vi "XX-孔数处理函数.vi"(0 "Image in":T2(plugin-control), 5 "参数输入":T1={"二值化参数"={"Lower value"=104.0, "Upper value"=255.0}, "Selection Values"=[{"Measurement Parameter"=35, "Range Lower Value"=1949.8375244140625, "Range Upper Value"=6069341.0, "Range"=FALSE, "Measurement Type"=FALSE}], "Selection Values2"=[{"Measurement Parameter"=19, "Range Lower Value"=98.7405776977539, "Range Upper Value"=135.92166137695312, "Range"=FALSE, "Measurement Type"=FALSE}]} {"Selection Values2"."Measurement Parameter" items=["Center of Mass X", "Center of Mass Y", "First Pixel X", "First Pixel Y", "Bounding Rect Left", "Bounding Rect Top", "Bounding Rect Right", "Bounding Rect Bottom", "Max Feret Diameter Start X", "Max Feret Diameter Start Y", "Max Feret Diameter End X", "Max Feret Diameter End Y", "Max Horiz. Segment Length Left", "Max Horiz. Segment Length Right", "Max Horiz. Segment Length Row", "-", "Bounding Rect Width", "Bounding Rect Height", "Bounding Rect Diagonal", "Perimeter", "Convex Hull Perimeter", "Holes' Perimeter", "Max Feret Diameter", "Equivalent Ellipse Major Axis", "Equivalent Ellipse Minor Axis", "Equivalent Ellipse Minor Axis (Feret)", "Equivalent Rect Long Side", "Equivalent Rect Short Side", "Equivalent Rect Diagonal", "Equivalent Rect Short Side (Feret)", "Average Horiz. Segment Length", "Average Vert. Segment Length", "Hydraulic Radius", "Waddel Disk Diameter", "-", "Area", "Holes' Area", "Particle & Holes' Area", "Convex Hull Area", "Image Area", "-", "Number of Holes", "Number of Horiz. Segments", "Number of Vert. Segments", "-", "Orientation", "Max Feret Diameter Orientation", "-", "% Area/Image Area", "% Area/(Particle & Holes' Area)", "Ratio of Equivalent Ellipse Axes", "Ratio of Equivalent Rect Sides", "-", "Elongation Factor", "Compactness Factor", "Heywood Circularity Factor", "Type Factor", "-", "Sum X", "Sum Y", "Sum XX", "Sum XY", "Sum YY", "Sum XXX", "Sum XXY", "Sum XYY", "Sum YYY", "-", "Moment of Inertia XX", "Moment of Inertia XY", "Moment of Inertia YY", "Moment of Inertia XXX", "Moment of Inertia XXY", "Moment of Inertia XYY", "Moment of Inertia YYY", "Norm. Moment of Inertia XX", "Norm. Moment of Inertia XY", "Norm. Moment of Inertia YY", "Norm. Moment of Inertia XXX", "Norm. Moment of Inertia XXY", "Norm. Moment of Inertia XYY", "Norm. Moment of Inertia YYY", "Hu Moment 1", "Hu Moment 2", "Hu Moment 3", "Hu Moment 4", "Hu Moment 5", "Hu Moment 6", "Hu Moment 7"]; "Selection Values"."Measurement Parameter" items=["Center of Mass X", "Center of Mass Y", "First Pixel X", "First Pixel Y", "Bounding Rect Left", "Bounding Rect Top", "Bounding Rect Right", "Bounding Rect Bottom", "Max Feret Diameter Start X", "Max Feret Diameter Start Y", "Max Feret Diameter End X", "Max Feret Diameter End Y", "Max Horiz. Segment Length Left", "Max Horiz. Segment Length Right", "Max Horiz. Segment Length Row", "-", "Bounding Rect Width", "Bounding Rect Height", "Bounding Rect Diagonal", "Perimeter", "Convex Hull Perimeter", "Holes' Perimeter", "Max Feret Diameter", "Equivalent Ellipse Major Axis", "Equivalent Ellipse Minor Axis", "Equivalent Ellipse Minor Axis (Feret)", "Equivalent Rect Long Side", "Equivalent Rect Short Side", "Equivalent Rect Diagonal", "Equivalent Rect Short Side (Feret)", "Average Horiz. Segment Length", "Average Vert. Segment Length", "Hydraulic Radius", "Waddel Disk Diameter", "-", "Area", "Holes' Area", "Particle & Holes' Area", "Convex Hull Area", "Image Area", "-", "Number of Holes", "Number of Horiz. Segments", "Number of Vert. Segments", "-", "Orientation", "Max Feret Diameter Orientation", "-", "% Area/Image Area", "% Area/(Particle & Holes' Area)", "Ratio of Equivalent Ellipse Axes", "Ratio of Equivalent Rect Sides", "-", "Elongation Factor", "Compactness Factor", "Heywood Circularity Factor", "Type Factor", "-", "Sum X", "Sum Y", "Sum XX", "Sum XY", "Sum YY", "Sum XXX", "Sum XXY", "Sum XYY", "Sum YYY", "-", "Moment of Inertia XX", "Moment of Inertia XY", "Moment of Inertia YY", "Moment of Inertia XXX", "Moment of Inertia XXY", "Moment of Inertia XYY", "Moment of Inertia YYY", "Norm. Moment of Inertia XX", "Norm. Moment of Inertia XY", "Norm. Moment of Inertia YY", "Norm. Moment of Inertia XXX", "Norm. Moment of Inertia XXY", "Norm. Moment of Inertia XYY", "Norm. Moment of Inertia YYY", "Hu Moment 1", "Hu Moment 2", "Hu Moment 3", "Hu Moment 4", "Hu Moment 5", "Hu Moment 6", "Hu Moment 7"]; "Selection Values"."Range Upper Value" format="%#_9f"}, 7 "图像处理开关":bool, 11 "error in":errorcluster) -> (4 "Image Out":T2(plugin-control), 10 "Particle Measurements (Pixels)":dbl[][](array[numeric]) format="%.2f", 15 "error out":errorcluster)   [LabVIEW 2017]
uses:
  Global System.vi
  <vilib>/vision/NI_Vision_Development_Module.lvlib
panel:
  out "millisecond timer value":u32
  in  "Range":cluster{"Lower value":sgl, "Upper value":sgl}={"Lower value"=104.0, "Upper value"=255.0}
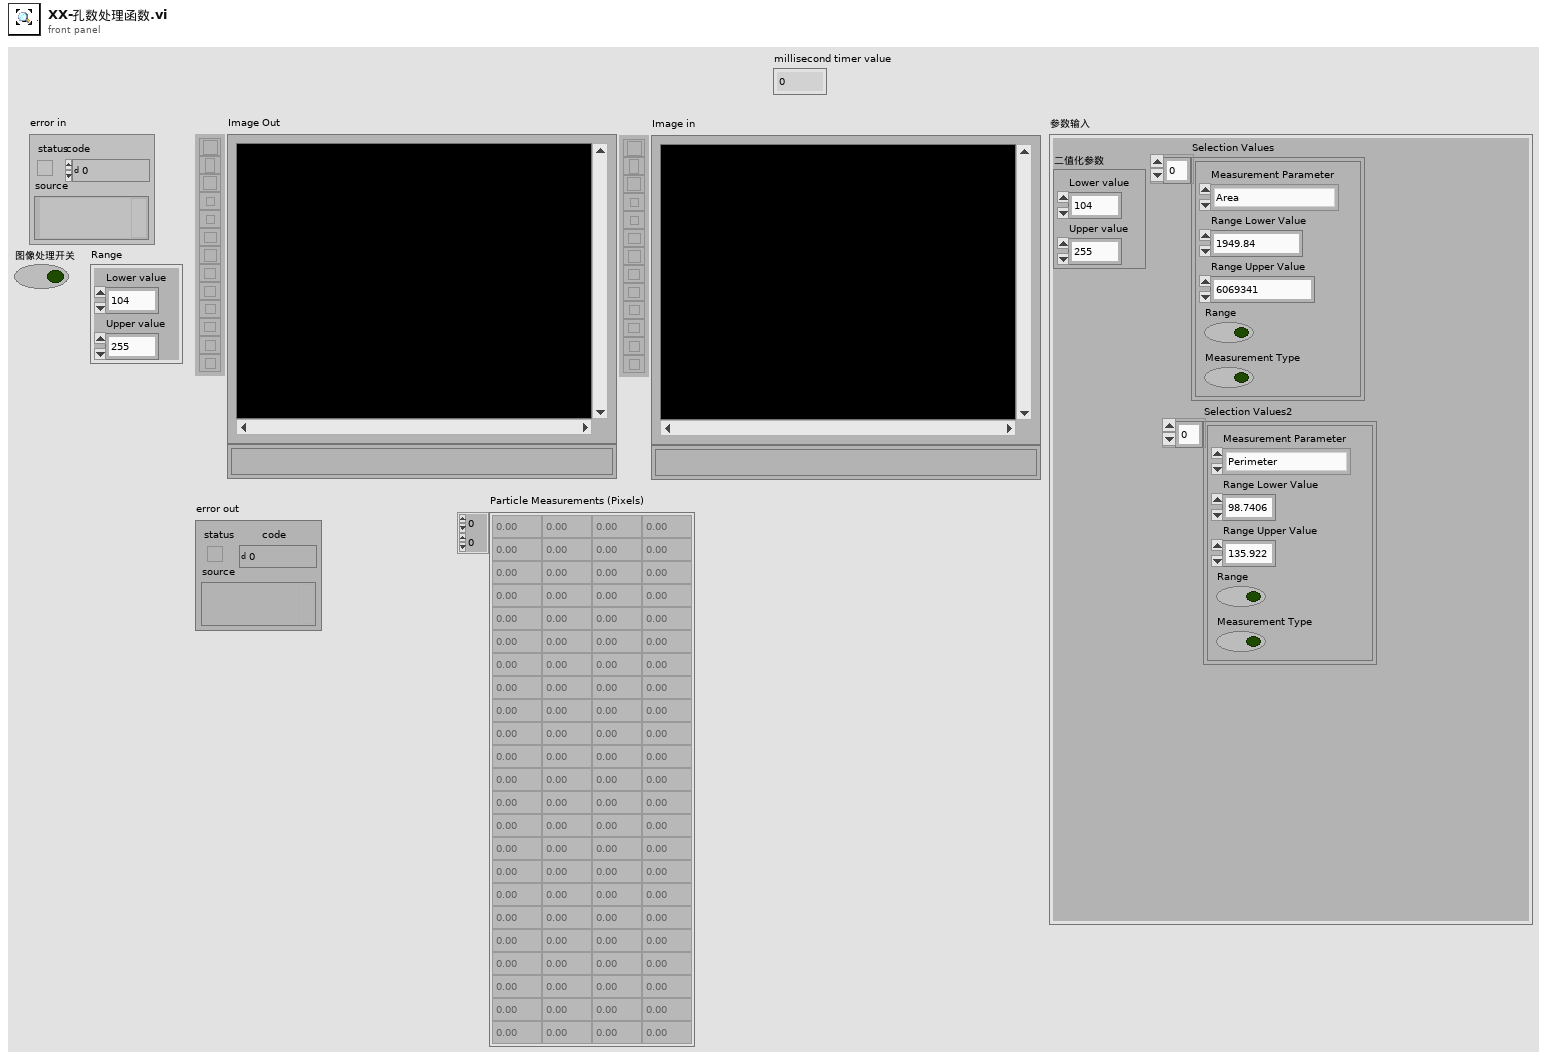
[diagram p1: front panel]
types:
  T1 = cluster{"二值化参数":cluster{"Lower value":sgl, "Upper value":sgl}, "Selection Values":cluster{"Measurement Parameter":i32, "Range Lower Value":dbl, "Range Upper Value":dbl, "Range":bool, "Measurement Type":bool}[], "Selection Values2":cluster{"Measurement Parameter":i32, "Range Lower Value":dbl, "Range Upper Value":dbl, "Range":bool, "Measurement Type":bool}[]}
  T2 = typedef "IMAQ Image.ctl" = refnum<image>
  T3 = cluster{"Measurement Parameter":i32, "Range Lower Value":dbl, "Range Upper Value":dbl, "Range":bool, "Measurement Type":bool}[]
  T4 = typedef "Image Type" = u32
  T5 = cluster{"histogram":u32[], "Minimal Value":sgl, "Maximal Value":sgl, "Starting Value":sgl, "Interval Width":sgl, "Mean Value":sgl, "Standard  Variation":sgl, "Area (pixels)":i32}
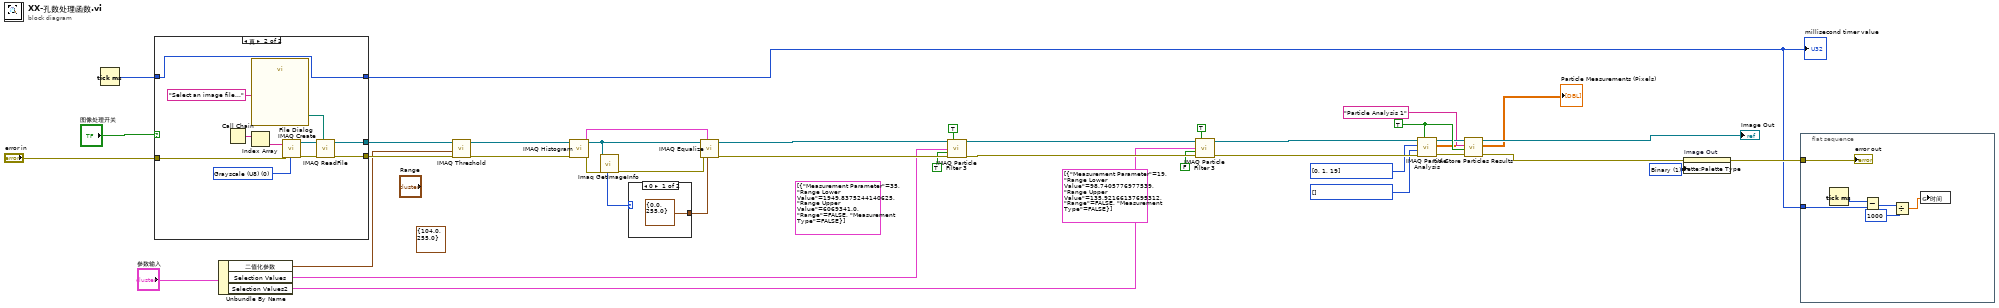
[diagram p0: block diagram]
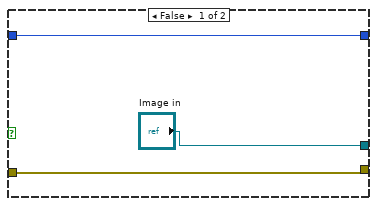
[diagram p2: hidden frame]
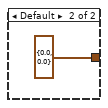
[diagram p3: hidden frame]
diagram:
  (unwired) cluster{"Lower value":sgl, "Upper value":sgl} {"Lower value"=104.0, "Upper value"=255.0} ("Range")
  w9 = u32 1 items=["Grayscale", "Binary", "Gradient", "Rainbow", "Temperature", "User Defined", "Binary 16 Bit", "Gradient 16 Bit", "Rainbow 16 Bit", "Temperature 16 Bit", "User Defined 16 Bit"] ("Palette Type")
  w18 = i32[] [] items=["Center of Mass X", "Center of Mass Y", "First Pixel X", "First Pixel Y", "Bounding Rect Left", "Bounding Rect Top", "Bounding Rect Right", "Bounding Rect Bottom", "Max Feret Diameter Start X", "Max Feret Diameter Start Y", "Max Feret Diameter End X", "Max Feret Diameter End Y", "Max Horiz. Segment Length Left", "Max Horiz. Segment Length Right", "Max Horiz. Segment Length Row", "-", "Bounding Rect Width", "Bounding Rect Height", "Bounding Rect Diagonal", "Perimeter", "Convex Hull Perimeter", "Holes' Perimeter", "Max Feret Diameter", "Equivalent Ellipse Major Axis", "Equivalent Ellipse Minor Axis", "Equivalent Ellipse Minor Axis (Feret)", "Equivalent Rect Long Side", "Equivalent Rect Short Side", "Equivalent Rect Diagonal", "Equivalent Rect Short Side (Feret)", "Average Horiz. Segment Length", "Average Vert. Segment Length", "Hydraulic Radius", "Waddel Disk Diameter", "-", "Area", "Holes' Area", "Particle & Holes' Area", "Convex Hull Area", "Image Area", "-", "Number of Holes", "Number of Horiz. Segments", "Number of Vert. Segments", "-", "Orientation", "Max Feret Diameter Orientation", "-", "% Area/Image Area", "% Area/(Particle & Holes' Area)", "Ratio of Equivalent Ellipse Axes", "Ratio of Equivalent Rect Sides", "-", "Elongation Factor", "Compactness Factor", "Heywood Circularity Factor", "Type Factor", "-", "Sum X", "Sum Y", "Sum XX", "Sum XY", "Sum YY", "Sum XXX", "Sum XXY", "Sum XYY", "Sum YYY", "-", "Moment of Inertia XX", "Moment of Inertia XY", "Moment of Inertia YY", "Moment of Inertia XXX", "Moment of Inertia XXY", "Moment of Inertia XYY", "Moment of Inertia YYY", "Norm. Moment of Inertia XX", "Norm. Moment of Inertia XY", "Norm. Moment of Inertia YY", "Norm. Moment of Inertia XXX", "Norm. Moment of Inertia XXY", "Norm. Moment of Inertia XYY", "Norm. Moment of Inertia YYY", "Hu Moment 1", "Hu Moment 2", "Hu Moment 3", "Hu Moment 4", "Hu Moment 5", "Hu Moment 6", "Hu Moment 7"] ("Real-World Measurements")
  w19 = i32[] [0, 1, 19] items=["Center of Mass X", "Center of Mass Y", "First Pixel X", "First Pixel Y", "Bounding Rect Left", "Bounding Rect Top", "Bounding Rect Right", "Bounding Rect Bottom", "Max Feret Diameter Start X", "Max Feret Diameter Start Y", "Max Feret Diameter End X", "Max Feret Diameter End Y", "Max Horiz. Segment Length Left", "Max Horiz. Segment Length Right", "Max Horiz. Segment Length Row", "-", "Bounding Rect Width", "Bounding Rect Height", "Bounding Rect Diagonal", "Perimeter", "Convex Hull Perimeter", "Holes' Perimeter", "Max Feret Diameter", "Equivalent Ellipse Major Axis", "Equivalent Ellipse Minor Axis", "Equivalent Ellipse Minor Axis (Feret)", "Equivalent Rect Long Side", "Equivalent Rect Short Side", "Equivalent Rect Diagonal", "Equivalent Rect Short Side (Feret)", "Average Horiz. Segment Length", "Average Vert. Segment Length", "Hydraulic Radius", "Waddel Disk Diameter", "-", "Area", "Holes' Area", "Particle & Holes' Area", "Convex Hull Area", "Image Area", "-", "Number of Holes", "Number of Horiz. Segments", "Number of Vert. Segments", "-", "Orientation", "Max Feret Diameter Orientation", "-", "% Area/Image Area", "% Area/(Particle & Holes' Area)", "Ratio of Equivalent Ellipse Axes", "Ratio of Equivalent Rect Sides", "-", "Elongation Factor", "Compactness Factor", "Heywood Circularity Factor", "Type Factor", "-", "Sum X", "Sum Y", "Sum XX", "Sum XY", "Sum YY", "Sum XXX", "Sum XXY", "Sum XYY", "Sum YYY", "-", "Moment of Inertia XX", "Moment of Inertia XY", "Moment of Inertia YY", "Moment of Inertia XXX", "Moment of Inertia XXY", "Moment of Inertia XYY", "Moment of Inertia YYY", "Norm. Moment of Inertia XX", "Norm. Moment of Inertia XY", "Norm. Moment of Inertia YY", "Norm. Moment of Inertia XXX", "Norm. Moment of Inertia XXY", "Norm. Moment of Inertia XYY", "Norm. Moment of Inertia YYY", "Hu Moment 1", "Hu Moment 2", "Hu Moment 3", "Hu Moment 4", "Hu Moment 5", "Hu Moment 6", "Hu Moment 7"] ("Pixel Measurements")
  w16 = TRUE ("Connectivity 4/8 (8)")
  (unwired) T3 [{"Measurement Parameter"=19, "Range Lower Value"=98.7405776977539, "Range Upper Value"=135.92166137695312, "Range"=FALSE, "Measurement Type"=FALSE}] ("Selection Values")
  (unwired) T3 [{"Measurement Parameter"=35, "Range Lower Value"=1949.8375244140625, "Range Upper Value"=6069341.0, "Range"=FALSE, "Measurement Type"=FALSE}] ("Selection Values")
  n1 = Tick Count (ms)() -> (millisecond timer value=w2:u32)
  n2 = case shown="真" "图像处理开关" {
    tunnel: [w40 w52] -> w38
    tunnel: "error in" -> [w40 w49]
    tunnel: ["Image in" w43] -> w36
    tunnel: w2 -> [w39 w42]
    tunnel: [w39 w42] -> w1
    frame False {
    }
    frame True {
      w44 = T4 0 items=["Grayscale (U8)", "Grayscale (I16)", "Grayscale (SGL)", "Complex (CSG)", "RGB (U32)", "HSL (U32)", "RGB (U64)", "Grayscale (U16)"] ("Image Type")
      n3 = Call Chain() -> (call chain=w48:string[])
      n4 = Index Array(array=w48) -> (element=w47:string)  [unwired: 1 in]
      n5 = call "File Dialog"("prompt"="Select an image file...") -> ("selected path"=w45:path)  [unwired: 6 in, 8 out]
      n6 = call "IMAQ Create"("Image Name"=w47, "Image Type"=w44, "error in (no error)"=w49) -> ("New Image"=w51:T2, "error out"=w50:errorcluster)  [unwired: 1 in, 1 out]
      n7 = call "IMAQ ReadFile"("File Path"=w45, "error in (no error)"=w50, "Image"=w51) -> ("error out"=w52:errorcluster, "Image Out"=w43:T2)  [unwired: 2 in, 5 out]
    }
  }
  "millisecond timer value" <- w1
  n8 = Unbundle By Name("参数输入") -> ("二值化参数"=w6:cluster{"Lower value":sgl, "Upper value":sgl}, "Selection Values"=w5:T3, "Selection Values2"=w4:T3)
  n9 = call "IMAQ Threshold"("error in (no error)"=w38, "Range"=w6, "Image Src"=w36) -> ("error out"=w35:errorcluster, "Image Dst Out"=w31:T2)  [unwired: 3 in, 4 out]
  n10 = call "IMAQ Histogram"("error in (no error)"=w35, "Image"=w31) -> ("error out"=w30:errorcluster, "Histogram Report"=w33:T5)  [unwired: 3 in, 5 out]
  n11 = call "Imaq GetImageInfo"("error in (no error)"=w30, "Image"=w31) -> ("error out"=w29:errorcluster, "Image Type"=w32:T4)  [unwired: 8 out]
  n12 = case "条件结构" shown="0" w32 {
    tunnel: [cluster{"Minimum":sgl, "Maximum":sgl} {"Minimum"=0.0, "Maximum"=255.0} ("Range") cluster{"Minimum":sgl, "Maximum":sgl} {"Minimum"=0.0, "Maximum"=0.0} ("Range")] -> w28
    frame 0 {
    }
    frame Default {
    }
  }
  n13 = call "IMAQ Equalize"("Range"=w28, "Histogram Report"=w33, "error in (no error)"=w29, "Image Src"=w31) -> ("error out"=w34:errorcluster, "Image Dst Out"=w24:T2)  [unwired: 2 in, 4 out]
  n14 = call "IMAQ Particle Filter 3"("Image Src"=w24, "Connectivity 4/8 (8)"=TRUE, "Selection Values"=w5, "Keep/Remove Particles (F)"=TRUE ("Keep/Remove Particles"), "error in (no error)"=w34) -> ("Image Dst Out"=w20:T2, "error out"=w25:errorcluster)  [unwired: 4 in, 5 out]
  n15 = call "IMAQ Particle Filter 3"("Image Src"=w20, "Connectivity 4/8 (8)"=TRUE, "Selection Values"=w4, "Keep/Remove Particles (F)"=FALSE ("Keep/Remove Particles"), "error in (no error)"=w25) -> ("Image Dst Out"=w17:T2, "error out"=w21:errorcluster)  [unwired: 4 in, 5 out]
  n16 = call "IMAQ Particle Analysis"("Connectivity 4/8 (8)"=w16, "error in (no error)"=w21, "Real-World Measurements"=w18, "Pixel Measurements"=w19, "Image"=w17) -> ("error out"=w13:errorcluster, "Particle Measurements (Pixels)"=→"Particle Measurements (Pixels)":dbl[][], "Image Out (duplicate)"=w15:T2)  [unwired: 4 out]
  n17 = call <vilib>:"IVA Store Particles Results.vi"("error in (no error)"=w13, "Connectivity 4/8 (8)"=w16, "Step Name"="Particle Analysis 1", "Image in"=w15) -> ("error out"=w12:errorcluster, "Image dup"=→"Image Out":T2)  [unwired: 6 out]
  n18 = property on="Image Out" class="ImageControl"(error in=w12, "Palette:Palette Type"=w9) -> (error out=w11:errorcluster)  [unwired: 1 in, 1 out]
  n19 = flat-sequence {
    tunnel: w11 -> [w60]
    tunnel: w1 -> [w58]
    frame #0 {
      n20 = Tick Count (ms)() -> (millisecond timer value=w59:u32)
      n21 = Subtract(x=w59, y=w58) -> (x-y=w57:u32)
      n22 = Divide(x=w57, y=u32 1000) -> (x/y=w55:dbl)
      n23 = global write "Global System.vi" "时间"(w55) -> ()
      "error out" <- w60
    }
  }
